vi "Add Service.vi"(6 "WebSocket Data Handler":refnum<class "WebSocket Connection Handler Msg.lvclass">, 7 "Receive Connection Enqueuer Handler":refnum<class "WebSocket Server-Service Enqueuer Msg.lvclass">, 8 "error in (no error)":errorcluster, 9 "Subscriber Enqueuer":refnum<class "Message Enqueuer.lvclass">, 10 "Service Name":string, 11 "WebSocket Server in":refnum<class "WebSocket Server.lvclass">) -> (0 "error out":errorcluster, 3 "WebSocket Server out":refnum<class "WebSocket Server.lvclass">)   [LabVIEW 2021, in "WebSocket Actors.lvlib" / "WebSocket Server.lvclass"]
doc: "This method will start a WebSocket service as specified by \"Service Name\". If the service is already running its enqueuer is returned to the subscriber, otherwise the service is also started, and the enqueuer returned."
uses:
  WebSocket Server.lvclass
  C:/Program Files/National Instruments/LabVIEW 2021/vi.lib/ActorFramework/Actor/Actor.lvclass
  <vilib>/ActorFramework/Message Enqueuer/Message Enqueuer.lvclass
  Abstract Messages/WebSocket Connection Handler Msg/WebSocket Connection Handler Msg.lvclass
  Abstract Messages/WebSocket Server-Service Enqueuer Msg/WebSocket Server-Service Enqueuer Msg.lvclass
  C:/Program Files/National Instruments/LabVIEW 2021/vi.lib/ActorFramework/Message/Message.lvclass
  WebSocket Server.lvclass/WebSocket Server.ctl
  WebSocket Service/WebSocket Service.lvclass
  WebSocket Service/WebSocket Service.lvclass/WebSocket Service.ctl
  Abstract Messages/WebSocket Server-Service Enqueuer Msg/WebSocket Server-Service Enqueuer Msg.lvclass/WebSocket Server-Service Enqueuer Msg.ctl
  <vilib>/ActorFramework/Message Enqueuer/Message Enqueuer.lvclass/Message Enqueuer.ctl
  <vilib>/ActorFramework/Actor/Actor.lvclass/Actor.ctl
  <vilib>/ActorFramework/Report Error Msg/Report Error Msg.lvclass/Report Error Msg.ctl
  WebSocket Service/properties/Write Subscriber Enqueuer.vi
  WebSocket Service/properties/Write WebSocket Data Handler.vi
  WebSocket Service/properties/Write Service Name.vi
  WebSocket Service/Write Keepalive.vi
  <vilib>/ActorFramework/Message Enqueuer/Enqueue.vi
  <vilib>/ActorFramework/Report Error Msg/Report Error Msg.lvclass
  <vilib>/Utility/LVClass/Get LV Class Name.vi
  <resource>/AFDebug/Generate Trace for Message.vi
  <vilib>/ActorFramework/Message Priority Queue/Priority Enqueue.vi
  <vilib>/Utility/error.llb/Error Cluster From Error Code.vi
  <vilib>/ErrorRing/Error Ring.xnode
  <vilib>/ActorFramework/Actor/Actor.lvclass
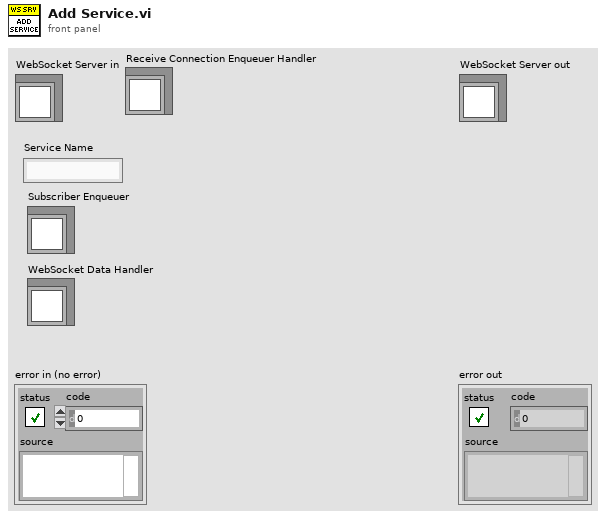
[diagram p1: front panel]
types:
  T1 = typedef "WebSocket Actors.lvlib/WebSocket Connection.lvclass/Keepalive.ctl" = cluster{"Enabled":bool, "Ping Interval (ms)":u32, "Ping Timeout (ms)":u32}
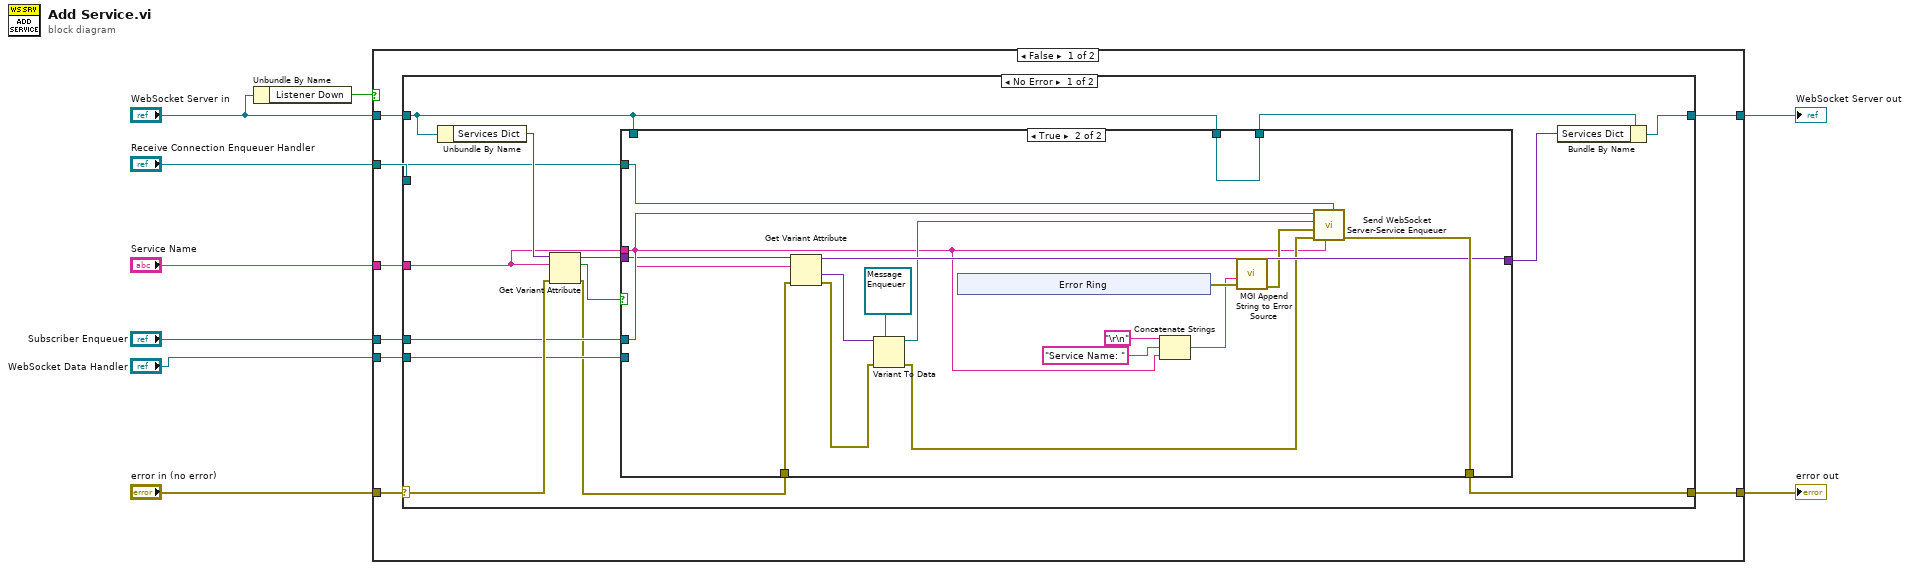
[diagram p0: block diagram]
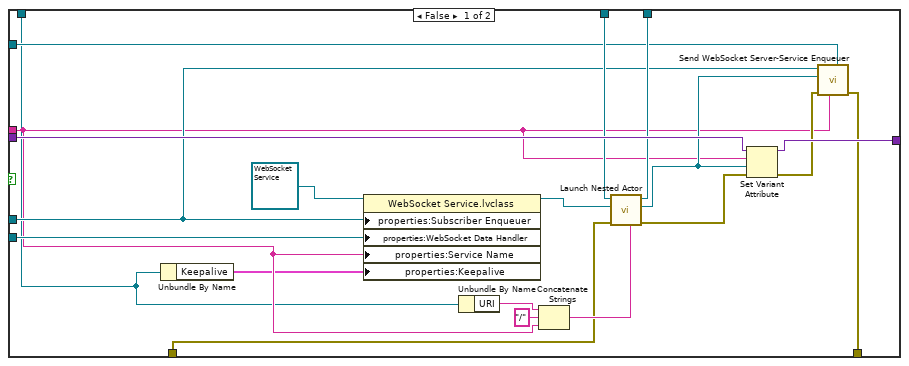
[diagram p2: hidden frame]
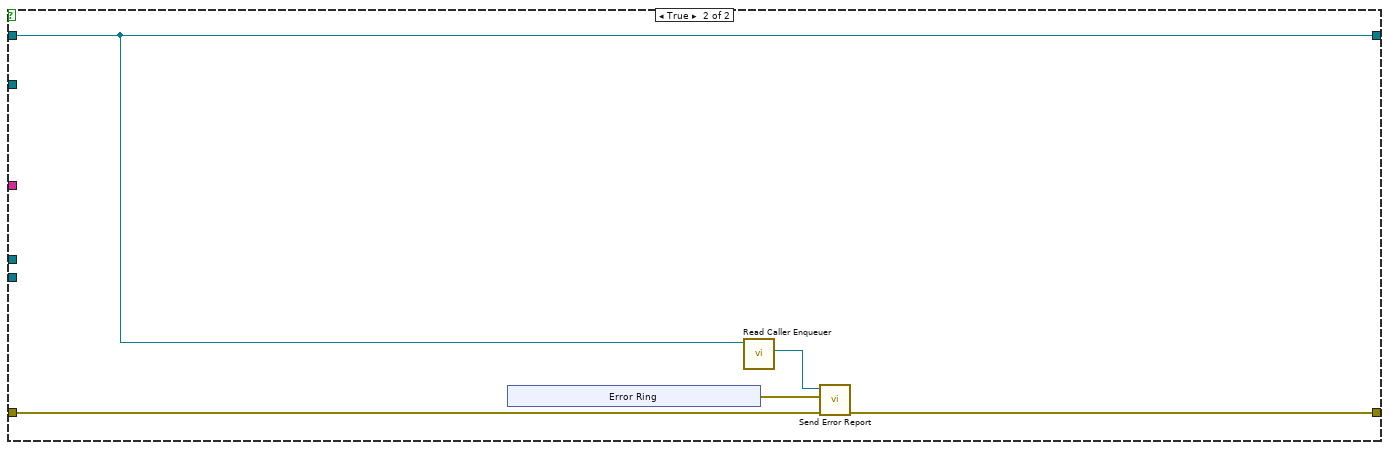
[diagram p4: hidden frame]
diagram:
  n1 = Unbundle By Name("WebSocket Server in") -> ("Listener Down"=w1:bool)
  n2 = case shown="False" w1 {
    tunnel: "error in (no error)" -> [w17 w78]
    tunnel: [w16 w77] -> w8
    tunnel: "WebSocket Server in" -> [w15 w76]
    tunnel: [w14 w76] -> w7
    tunnel: "Service Name" -> [w13 _]
    tunnel: "Subscriber Enqueuer" -> [w12 _]
    tunnel: "WebSocket Data Handler" -> [w11 _]
    tunnel: "Receive Connection Enqueuer Handler" -> [w10 _]
    frame False {
      n3 = case shown="No Error" w17 {
        selector: w17 -> [w28 w75]
        tunnel: [w25 w75] -> w16
        tunnel: [w31 w74] -> w14
        tunnel: w15 -> [w21 w74]
        tunnel: w13 -> [w27 _]
        tunnel: w12 -> [w22 _]
        tunnel: w11 -> [w20 _]
        tunnel: w10 -> [w19 _]
        frame No Error {
          n4 = Unbundle By Name(w21) -> ("Services Dict"=w30:variant)
          n5 = Get Variant Attribute(Variant=w30, name=w27, error in=w28) -> (duplicate Variant=w24:variant, found=w29:bool, error out=w18:errorcluster)  [unwired: 1 in, 1 out]
          n6 = case shown="True" w29 {
            tunnel: w27 -> [w34 w52]
            tunnel: [w42 w69] -> w26
            tunnel: [w39 w66] -> w25
            tunnel: w24 -> [w51 w65]
            tunnel: [w50 w64] -> w23
            tunnel: w21 -> [w33 _]
            tunnel: w22 -> [w37 w67]
            tunnel: w21 -> [w43 w69]
            tunnel: w20 -> [w41 _]
            tunnel: w19 -> [w36 w68]
            tunnel: w18 -> [w35 w63]
            frame False {
              n7 = Unbundle By Name(w33) -> ("Keepalive"=w32:T1)
              n8 = property class="WebSocket Service.lvclass"(reference=refnum<class "WebSocket Service.lvclass"> refnum ("WebSocket Actor.lvlib:WebSocket Service Actor.lvclass"), "properties:Subscriber Enqueuer"=w37, "properties:WebSocket Data Handler"=w41, "properties:Service Name"=w34, "properties:Keepalive"=w32) -> (reference out=w44:refnum<class "WebSocket Service.lvclass">)  [unwired: 1 in, 1 out]
              n9 = Unbundle By Name(w33) -> ("URI"=w46:string)
              n10 = Concatenate Strings(w46, "/" ("string"), w34) -> (w48:string)
              n11 = call <vilib>:"Launch Nested Actor.vi"("Debug Alias"=w48, "error in (no error)"=w35, "Nested Actor"=w44, "Caller Actor in"=w43) -> ("error out"=w45:errorcluster, "Nested Actor's Enqueuer"=w38:refnum<class "Message Enqueuer.lvclass">, "Caller Actor out"=w42:refnum<class "WebSocket Server.lvclass">)  [unwired: 5 in]
              n12 = Set Variant Attribute(Variant=w51, name=w34, value=w38, error in=w45) -> (Variant out=w50:variant, error out=w40:errorcluster)  [unwired: 1 out]
              n13 = call "Send WebSocket Server-Service Enqueuer.vi"("Receive Service/Server Enqueuer Handler"=w36, "Service Name"=w34, "error in (no error)"=w40, "WebSocket Server/Service Enqueuer"=w38, "Message Enqueuer"=w37) -> ("error out"=w39:errorcluster)  [unwired: 5 in, 1 out]
            }
            frame True {
              n14 = Get Variant Attribute(Variant=w65, name=w52, error in=w63) -> (duplicate Variant=w64:variant, value=w59:variant, error out=w61:errorcluster)  [unwired: 1 in, 1 out]
              n15 = Variant To Data(error in=w61, type=refnum<class "Message Enqueuer.lvclass"> refnum ("WebSocket Service Enqueuer"), Variant=w59) -> (data=w58:refnum<class "Message Enqueuer.lvclass">, error out=w60:errorcluster)
              n16 = xnode "Error Ring"() -> ("error out"=w55:errorcluster)
              n17 = Concatenate Strings("\r\n", "Service Name: " ("string"), w52) -> (w53:string)
              n18 = call <userlib>:"MGI Append String to Error Source.vi"("Error In"=w55, "String to Append"=w53) -> ("Error Out"=w54:errorcluster)  [unwired: 9 in]
              n19 = call "Send WebSocket Server-Service Enqueuer.vi"("Receive Service/Server Enqueuer Handler"=w68, "Service Name"=w52, "error in (no error)"=w60, "Error"=w54, "WebSocket Server/Service Enqueuer"=w58, "Message Enqueuer"=w67) -> ("error out"=w66:errorcluster)  [unwired: 4 in, 1 out]
            }
          }
          n20 = Bundle By Name(cluster=w26, "Services Dict"=w23) -> (w31:refnum<class "WebSocket Server.lvclass">)
        }
        frame Error {
        }
      }
    }
    frame True {
      n21 = xnode "Error Ring"() -> ("error out"=w80:errorcluster)
      n22 = call <vilib>:"Read Caller Enqueuer.vi"("Actor"=w76) -> ("Caller Enqueuer"=w79:refnum<class "Message Enqueuer.lvclass">)  [unwired: 10 in]
      n23 = call <vilib>:"Send Error Report.vi"("error in (no error)"=w78, "Error From Sender"=w80, "Message Enqueuer"=w79) -> ("error out"=w77:errorcluster)  [unwired: 8 in]
    }
  }
  "error out" <- w8
  "WebSocket Server out" <- w7
